vi "AMI1700eth_meas_n2_lev.vi"(8 "error in":errorcluster, 11 "conn_id_in":refnum<k5>) -> (0 "error out":errorcluster, 2 "level":dbl, 3 "conn_id_out":refnum<k5>, 4 "status":bool)   [LabVIEW 2019]
panel:
  out "string 1":string
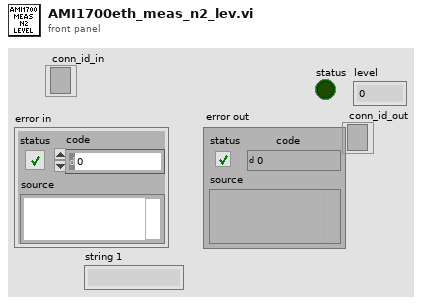
[diagram p1: front panel]
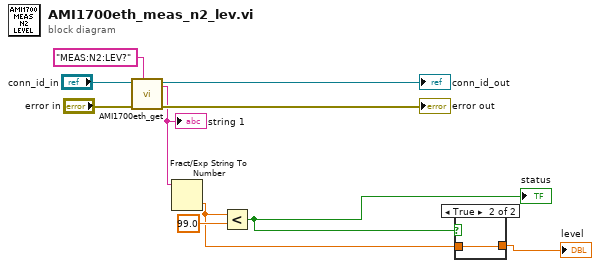
[diagram p0: block diagram]
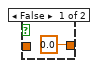
[diagram p2: hidden frame]
diagram:
  n1 = call "AMI1700eth_get.vi"("command"="MEAS:N2:LEV?" ("string"), "error in"="error in", "conn_id_in"="conn_id_in") -> ("error out"=→"error out":errorcluster, "conn_id_out"=→"conn_id_out":refnum<k5>, "string"=w6:string)  [unwired: 5 in, 1 out]
  "string 1" <- w6
  n2 = Fract/Exp String To Number(string=w6) -> (number=w4:dbl)  [unwired: 3 in, 1 out]
  n3 = Less?(x=w4, y=99.0) -> (x < y?=w5:bool)
  "status" <- w5
  n4 = case shown="True" w5 {
    tunnel: [0.0 w12] -> w3
    tunnel: w4 -> [_ w12]
    frame False {
    }
    frame True {
    }
  }
  "level" <- w3
